vi "JAUS Local WP to GPS WP.vi"(1 "Initial Yaw":dbl, 2 "Starting GPS WP":T1 {"Longitude" format="%#_14g"; "Latitude" format="%#_14g"}, 3 "LocalPose":T2, 4 "Local Waypoint List":T4[](array[typedef])) -> (0 "GPS WP List Out":T1[](array[typedef]) {"Longitude" format="%#_14g"; "Latitude" format="%#_14g"})   [LabVIEW 2009]
uses:
  JAUS/Support Files/ElementRec.ctl
  JAUS/Support Files/LocalWaypointRec.ctl
  JAUS/Support Files/LocalPose.ctl
  JAUS/Support Files/TimeRec.ctl
  TypeDefs/Sensor TypeDefs/GPS Data.ctl
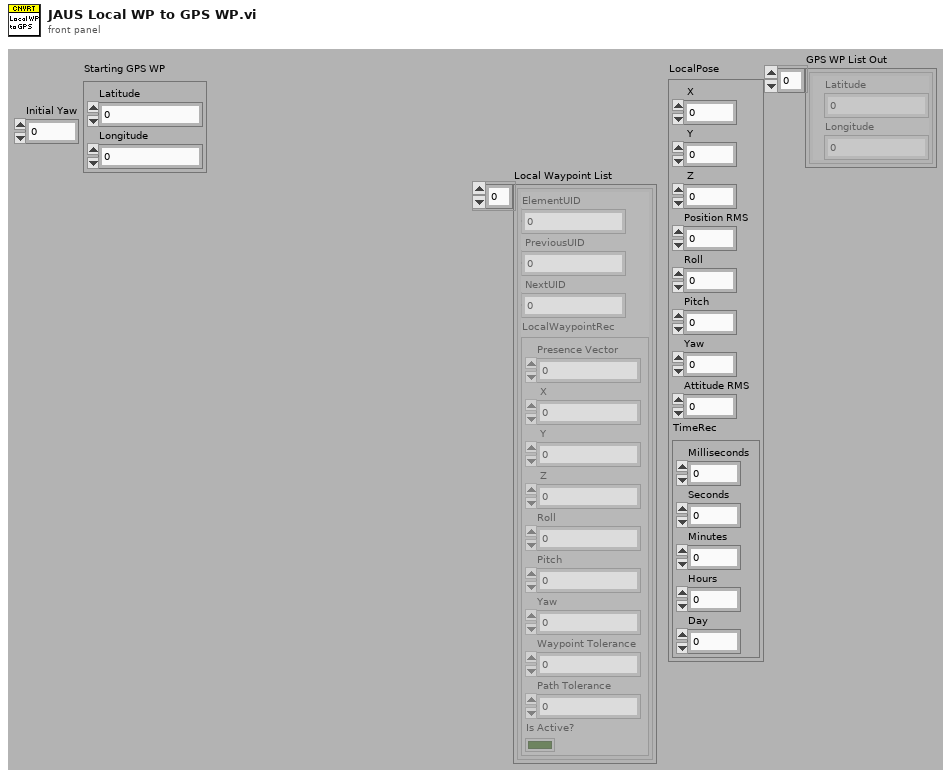
[diagram p1: front panel]
types:
  T1 = typedef "GPS Data.ctl" = cluster{"Latitude":dbl, "Longitude":dbl}
  T2 = typedef "LocalPose.ctl" = cluster{" X":dbl, " Y":dbl, " Z":dbl, "Position RMS":dbl, "Roll":dbl, "Pitch":dbl, "Yaw":dbl, "Attitude RMS":dbl, "TimeRec":T3}
  T3 = typedef "TimeRec.ctl" = cluster{"Milliseconds":u32, "Seconds":u32, "Minutes":u32, "Hours":u32, "Day":u32}
  T4 = typedef "ElementRec.ctl" = cluster{"ElementUID":u16, " PreviousUID":u16, " NextUID":u16, "LocalWaypointRec":T5}
  T5 = typedef "LocalWaypointRec.ctl" = cluster{"Presence Vector":u8, " X":dbl, " Y":dbl, " Z":dbl, "Roll":dbl, "Pitch":dbl, "Yaw":dbl, "Waypoint Tolerance":dbl, "Path Tolerance":dbl, "Is Active?":bool}
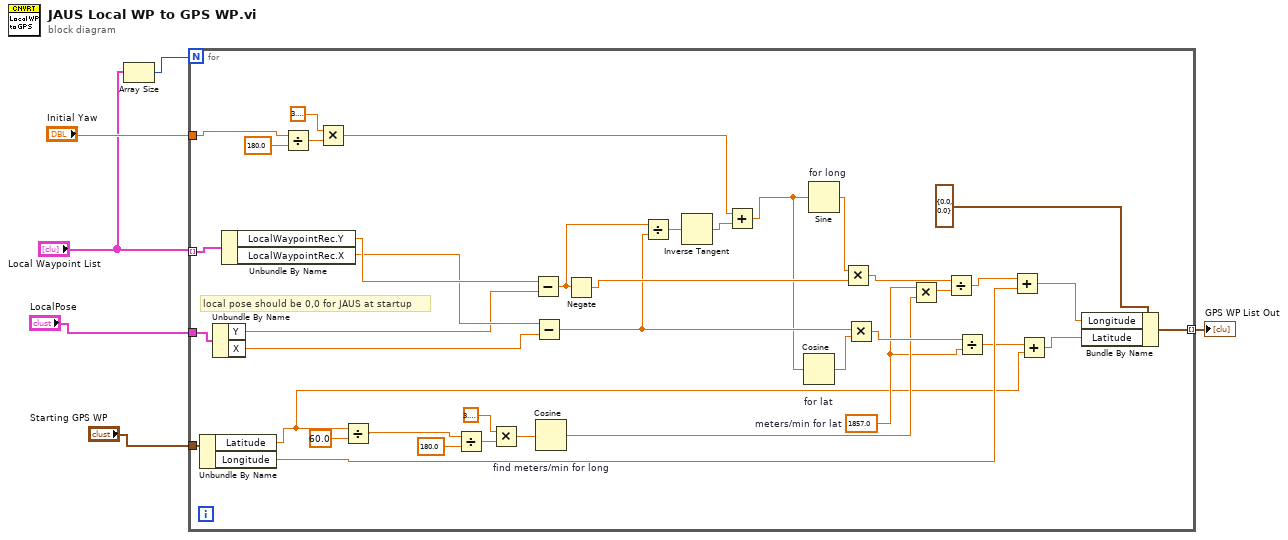
[diagram p0: block diagram]
diagram:
  n1 = Array Size(array="Local Waypoint List") -> (size(s)=w5:i32)
  n2 = for {
    N: w5 -> [_]
    tunnel: "Local Waypoint List" -> [w45] mode=indexing
    tunnel: "Initial Yaw" -> [w35]
    tunnel: "LocalPose" -> [w44]
    tunnel: "Starting GPS WP" -> [w24]
    tunnel: [w7] -> w1 mode=indexing
    w15 = 1857.0  # meters/min for lat
    # "local pose should be 0,0 for JAUS at startup"
    n3 = Unbundle By Name(w24) -> ("Latitude"=w13:dbl, "Longitude"=w14:dbl)
    n4 = Unbundle By Name(w44) -> ("Y"=w41:dbl, "X"=w40:dbl)
    n5 = Unbundle By Name(w45) -> ("LocalWaypointRec.Y"=w43:dbl, "LocalWaypointRec.X"=w42:dbl)
    n6 = Divide(x=w35, y=180.0) -> (x/y=w37:dbl)
    n7 = Multiply(x=3.141592653589793, y=w37) -> (x*y=w30:dbl)
    n8 = Divide(x=w13, y=60.0) -> (x/y=w19:dbl)
    n9 = Divide(x=w19, y=180.0) -> (x/y=w21:dbl)
    n10 = Multiply(x=3.141592653589793, y=w21) -> (x*y=w18:dbl)
    n11 = Subtract(x=w43, y=w41) -> (x-y=w34:dbl)
    n12 = Subtract(x=w42, y=w40) -> (x-y=w33:dbl)
    n13 = Cosine "find meters/min for long"(x=w18) -> (cos(x)=w16:dbl)
    n14 = Negate(x=w34) -> (-x=w39:dbl)
    n15 = Divide(x=w34, y=w33) -> (x/y=w32:dbl)
    n16 = Inverse Tangent(1:w32) -> (0:w31:dbl)
    n17 = Add(x=w30, y=w31) -> (x+y=w29:dbl)
    n18 = Cosine "for lat"(x=w29) -> (cos(x)=w27:dbl)
    n19 = Sine "for long"(x=w29) -> (sin(x)=w28:dbl)
    n20 = Multiply(x=w28, y=w39) -> (x*y=w26:dbl)
    n21 = Multiply(x=w33, y=w27) -> (x*y=w25:dbl)
    n22 = Multiply(x=w15, y=w16) -> (x*y=w17:dbl)
    n23 = Divide(x=w26, y=w17) -> (x/y=w11:dbl)
    n24 = Divide(x=w25, y=w15) -> (x/y=w12:dbl)
    n25 = Add(x=w11, y=w14) -> (x+y=w8:dbl)
    n26 = Add(x=w12, y=w13) -> (x+y=w9:dbl)
    n27 = Bundle By Name(cluster=T1 {"Latitude"=0.0, "Longitude"=0.0} ("Starting GPS WP 2"), "Longitude"=w8, "Latitude"=w9) -> (w7:T1)
  }
  "GPS WP List Out" <- w1
